vi "Initial_Lootkup Table - Y Step.vi"() -> ()   [LabVIEW 2015]
uses:
  <vilib>/Analysis/NI_AALBase.lvlib
panel:
  out "波形图":dbl[](graph)
  out "Init Data Out":i16[](array[numeric])
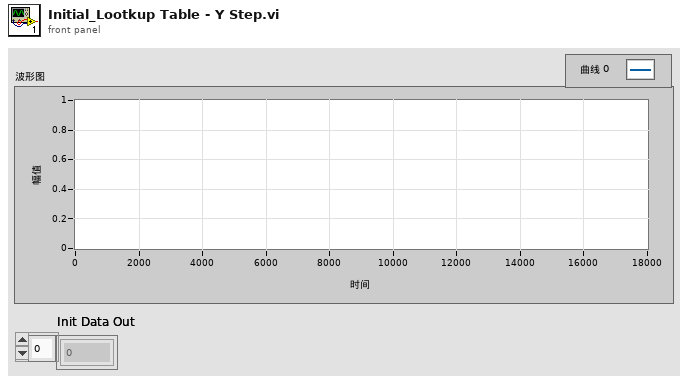
[diagram p1: front panel]
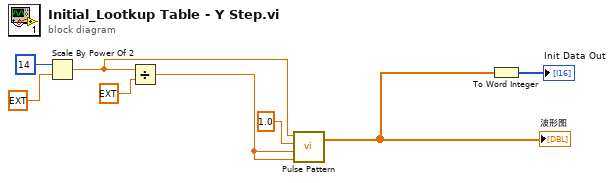
[diagram p0: block diagram]
diagram:
  n1 = Scale By Power Of 2(n=i16 14, x=ext 1.0) -> (x*2^n=w2:ext)
  n2 = Divide(x=w2, y=ext 2.0) -> (x/y=w1:ext)
  n3 = call <vilib>:"Pulse Pattern.vi"("width"=w1, "delay"=w1, "amplitude"=1.0, "samples"=w2) -> ("Pulse Pattern"=w3:dbl[])  [unwired: 1 out]
  "波形图" <- w3
  n4 = To Word Integer(number=w3) -> (16bit integer=→"Init Data Out":i16[])
